vi "Inverse Quaternion.vi"(0 "quaternion":T1) -> (2 "inverse":T1)   [LabVIEW 2017, in "NI_Kinematics.lvlib"]
doc: "Returns the inverse of a quaternion. \n\n<B>.m file:</B> inv"
uses:
  <vilib>/robotics/Kinematics/NI_Kinematics.lvlib
  <vilib>/robotics/Kinematics/Quaternion.ctl
  <vilib>/Analysis/baseanly.llb/Real Dot Product.vi
  <vilib>/Analysis/NI_AALBase.lvlib
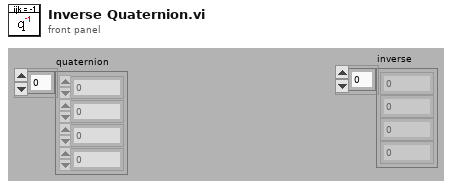
[diagram p1: front panel]
types:
  T1 = typedef "NI_Kinematics.lvlib/Quaternion.ctl" = dbl[]
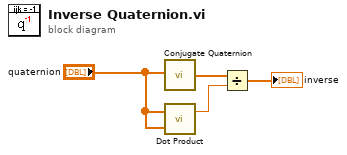
[diagram p0: block diagram]
diagram:
  n1 = call <vilib>:"Conjugate Quaternion.vi"("quaternion"="quaternion") -> ("conjugate"=w2:T1)
  n2 = call-poly <vilib>:"Dot Product.vi"("Y Vector"="quaternion", "X Vector"="quaternion") -> ("X * Y"=w1:dbl)  [unwired: 1 out]
  n3 = Divide(x=w2, y=w1) -> (x/y=→"inverse":T1)
